vi "Read Count.vi"(8 "error in (no error)":errorcluster, 11 "String Database in":refnum<class "String Database.lvclass">=refnum) -> (0 "error out":errorcluster, 2 "Count":i32, 3 "String Database out":refnum<class "String Database.lvclass">)   [LabVIEW 2018, in "String Database.lvlib" / "String Database.lvclass"]
uses:
  String Database.lvclass
  String Database.lvclass/String Database.ctl
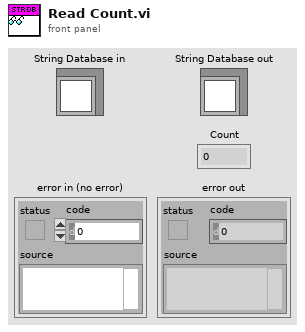
[diagram p1: front panel]
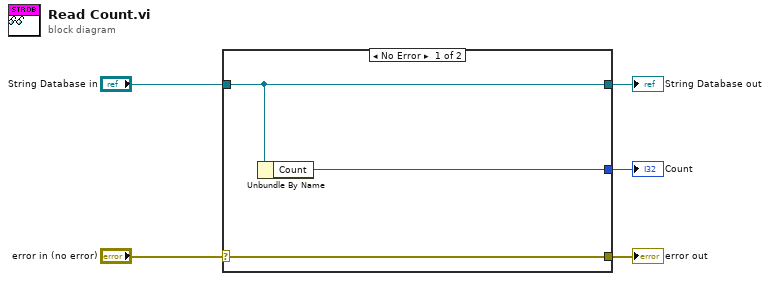
[diagram p0: block diagram]
diagram:
  n1 = case shown="No Error" "error in (no error)" {
    selector: "error in (no error)" -> [w8 w9]
    tunnel: [w8 w9] -> w4
    tunnel: [w7 w10] -> w2
    tunnel: "String Database in" -> [w7 w10]
    tunnel: [w6 _] -> w1
    frame No Error {
      n2 = Unbundle By Name(w7) -> ("Count"=w6:i32)
    }
    frame Error {
    }
  }
  "error out" <- w4
  "String Database out" <- w2
  "Count" <- w1
